vi "iWorx Chart Autoscale.vi"(7 "Selection Chart":refnum<vi>, 8 "Error In":errorcluster, 9 "Rounding Multiple (10)":dbl=10.0, 10 "Padding (10%)":dbl=10.0, 11 "Min Range (1)":dbl=1.0) -> (0 "error out":errorcluster, 2 "Min_Rounded":dbl, 3 "Max_Rounded":dbl)   [LabVIEW 2012]
doc: "This subVI is designed to autoscale a waveform chart based on the data that is currently visible on the chart."
uses:
  <vilib>/Utility/miscctls.llb/LVRangeTypeDef.ctl
panel:
  out "Output Scaling":T1
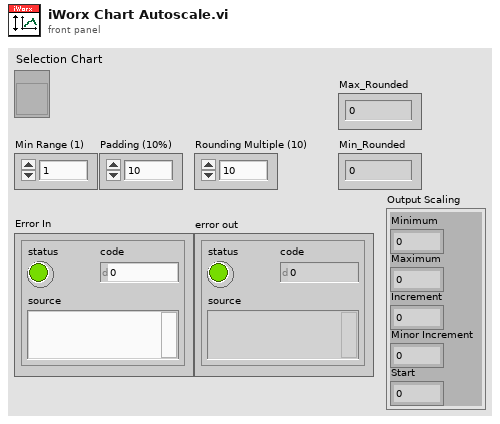
[diagram p1: front panel]
types:
  T1 = typedef "LVRangeTypeDef.ctl" = cluster{"Minimum":dbl, "Maximum":dbl, "Increment":dbl, "Minor Increment":dbl, "Start":dbl}
  T2 = cluster{"Minimum":bool, "Maximum":bool, "Increment":bool, "Minor Increment":bool, "Start":bool}
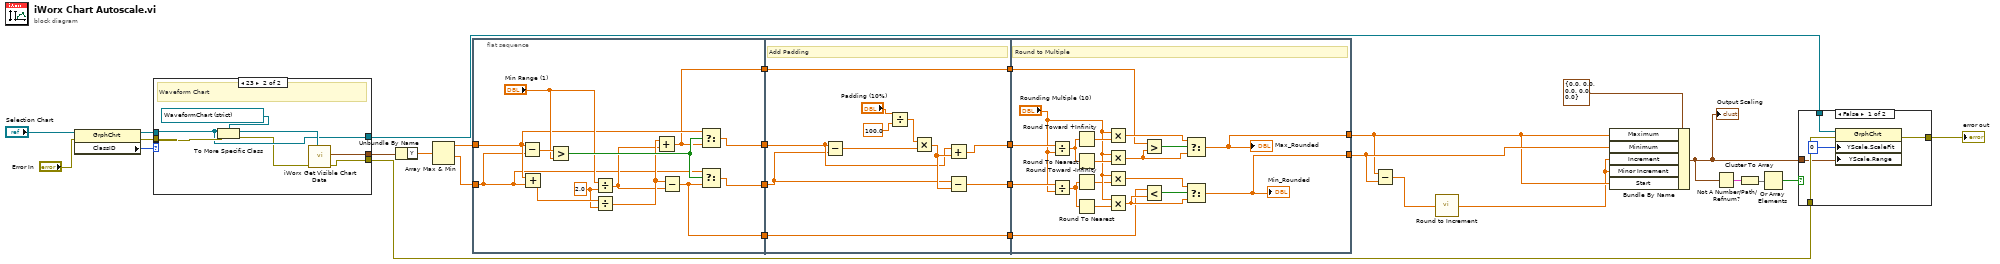
[diagram p0: block diagram]
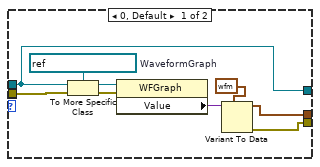
[diagram p2: hidden frame]
diagram:
  n1 = property class="GrphChrt"(reference="Selection Chart", error in="Error In") -> (reference out=w3:refnum<vi>, error out=w1:errorcluster, "ClassID"=w2:u32)
  n2 = case shown="23" w2 {
    tunnel: [w31 w40] -> w12
    tunnel: [w32 w45] -> w11
    tunnel: [w30 w41] -> w5
    tunnel: w3 -> [w30 w41]
    tunnel: w1 -> [_ w44]
    tunnel: w1 -> [w38 _]
    frame 0, Default {
      w37 = refnum<vi> refnum  # WaveformGraph
      n3 = To More Specific Class(target class=w37, reference=w30, error in=w38) -> (specific class reference=w36:refnum<vi>, error out=w35:errorcluster)
      n4 = property class="WFGraph"(reference=w36, error in=w35) -> ("Value"=w34:variant)  [unwired: 2 out]
      n5 = Variant To Data(type=waveform(dbl) {"t0"=timestamp(0 s since 1904-01-01), "dt"=1.0, "Y"=[]} ("Waveform"), Variant=w34) -> (data=w32:waveform(dbl), error out=w31:errorcluster)  [unwired: 1 in]
    }
    frame 23 {
      # "Waveform Chart"
      n6 = To More Specific Class(target class=refnum<vi> refnum ("Selection Chart"), reference=w41, error in=w44) -> (specific class reference=w43:refnum<vi>, error out=w39:errorcluster)
      n7 = call "iWorx Get Visible Chart Data.vi"("Selection Chart"=w43, "Error In"=w39) -> ("Error Out"=w40:errorcluster, "Waveform out"=w45:waveform(dbl))  [unwired: 7 in, 1 out]
    }
  }
  n8 = Unbundle By Name(w11) -> ("Y"=w17:dbl[])
  n9 = Array Max & Min(array=w17) -> (max value=w29:dbl, min value=w28:dbl)  [unwired: 2 out]
  n10 = flat-sequence {
    tunnel: w28 -> [w47]
    tunnel: w29 -> [w52]
    tunnel: [w51] -> w27
    tunnel: [w50] -> w26
    tunnel: [w49] -> w25
    tunnel: [w48] -> w24
    tunnel: [w62] -> w23
    tunnel: [w61] -> w22
    tunnel: w27 -> [w64]
    tunnel: w26 -> [w63]
    tunnel: [w60] -> w21
    tunnel: w25 -> [w60]
    tunnel: [w59] -> w20
    tunnel: w24 -> [w59]
    tunnel: w23 -> [w88]
    tunnel: w21 -> [w73]
    tunnel: w20 -> [w72]
    tunnel: w22 -> [w87]
    tunnel: [w71] -> w15
    tunnel: [w70] -> w18
    frame #0 {
      w46 = 2.0 ("y")
      n11 = Subtract(x=w52, y=w47) -> (x-y=w58:dbl)
      n12 = Add(x=w52, y=w47) -> (x+y=w56:dbl)
      n13 = Greater?(x=w58, y="Min Range (1)") -> (0:w57:bool)
      n14 = Divide(x="Min Range (1)", y=w46) -> (x/y=w53:dbl)
      n15 = Divide(x=w56, y=w46) -> (x/y=w54:dbl)
      n16 = Add(x=w54, y=w53) -> (x+y=w49:dbl)
      n17 = Subtract(x=w54, y=w53) -> (x-y=w48:dbl)
      n18 = Select(t=w52, s=w57, f=w49) -> (s? t:f=w51:dbl)
      n19 = Select(t=w47, s=w57, f=w48) -> (s? t:f=w50:dbl)
    }
    frame #1 {
      # "Add Padding"
      n20 = Subtract(x=w64, y=w63) -> (x-y=w66:dbl)
      n21 = Divide(x="Padding (10%)", y=100.0) -> (x/y=w67:dbl)
      n22 = Multiply(x=w67, y=w66) -> (x*y=w65:dbl)
      n23 = Add(x=w64, y=w65) -> (x+y=w62:dbl)
      n24 = Subtract(x=w63, y=w65) -> (x-y=w61:dbl)
    }
    frame #2 {
      # "Round to Multiple"
      n25 = Divide(x=w88, y="Rounding Multiple (10)") -> (x/y=w86:dbl)
      n26 = Divide(x=w87, y="Rounding Multiple (10)") -> (x/y=w85:dbl)
      n27 = Round Toward +Infinity(x=w86) -> (ceil(x): smallest int >= x=w82:dbl)
      n28 = Round To Nearest(number=w86) -> (nearest integer value=w81:dbl)
      n29 = Round Toward -Infinity(1:w85) -> (0:w76:dbl)
      n30 = Round To Nearest(number=w85) -> (nearest integer value=w78:dbl)
      n31 = Multiply(x="Rounding Multiple (10)", y=w82) -> (x*y=w80:dbl)
      n32 = Multiply(x="Rounding Multiple (10)", y=w81) -> (x*y=w79:dbl)
      n33 = Multiply(x="Rounding Multiple (10)", y=w76) -> (x*y=w75:dbl)
      n34 = Multiply(x="Rounding Multiple (10)", y=w78) -> (x*y=w74:dbl)
      n35 = Greater?(x=w73, y=w79) -> (0:w84:bool)
      n36 = Less?(x=w72, y=w74) -> (x < y?=w83:bool)
      n37 = Select(t=w80, s=w84, f=w79) -> (s? t:f=w71:dbl)
      "Max_Rounded" <- w71
      n38 = Select(t=w75, s=w83, f=w74) -> (s? t:f=w70:dbl)
      "Min_Rounded" <- w70
    }
  }
  n39 = Subtract(x=w15, y=w18) -> (x-y=w14:dbl)
  n40 = call "Round to Increment.vi"("Input"=w14) -> ("Output"=w13:dbl)
  n41 = Bundle By Name(cluster=T1 {"Minimum"=0.0, "Maximum"=0.0, "Increment"=0.0, "Minor Increment"=0.0, "Start"=0.0} ("Y Scale.Range"), "Maximum"=w15, "Minimum"=w18, "Increment"=w13, "Minor Increment"=w13, "Start"=w15) -> (w10:T1)
  "Output Scaling" <- w10
  n42 = Not A Number/Path/Refnum?(number/path/refnum=w10) -> (NaN/Path/Refnum?=w9:T2)
  n43 = Cluster To Array(cluster=w9) -> (array=w8:bool[])
  n44 = Or Array Elements(Boolean array=w8) -> (logical OR=w7:bool)
  n45 = case shown="False" w7 {
    tunnel: [w93 w94] -> w16
    tunnel: w12 -> [w91 w94]
    tunnel: w5 -> [w90 _]
    tunnel: w10 -> [w89 _]
    frame False {
      n46 = property class="GrphChrt"(reference=w90, error in=w91, "YScale.ScaleFit"=u8 0 ("Y Scale.Scale Fit"), "YScale.Range"=w89) -> (error out=w93:errorcluster)  [unwired: 1 out]
    }
    frame True {
      # "NaN\nDo not scale"
    }
  }
  "error out" <- w16
